vi "Coord window-FOV multiplier.vi"(11 "Absolute maximum coordinate":dbl) -> (3 "Field of view multiplier":sgl)   [LabVIEW 2013]
uses:
  <vilib>/gmath/NI_Gmath.lvlib
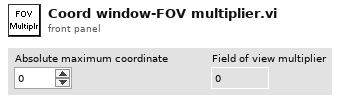
[diagram p1: front panel]
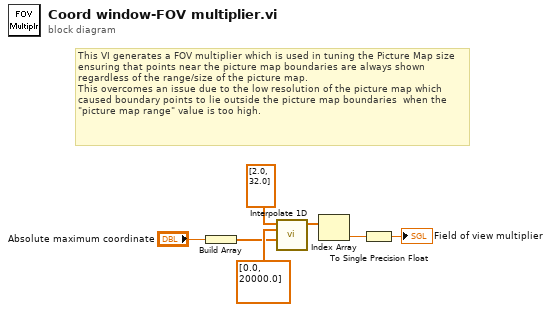
[diagram p0: block diagram]
diagram:
  # "This VI generates a FOV multiplier which is used in tuning the Picture Map size ensuring that points near the picture map boundaries are always shown regardless of the range/size of the picture map.\nThis overcomes an issue due to the low resolution of the picture map which caused boundary points to lie outside the picture map boundaries  when the \"picture map range\" value is too high."
  n1 = Build Array("Absolute maximum coordinate") -> (w4:dbl[])
  n2 = call <vilib>:"Interpolate 1D.vi"("xi"=w4, "X"=dbl[] [0.0, 20000.0] ("Y"), "Y"=dbl[] [2.0, 32.0]) -> ("yi"=w6:dbl[])  [unwired: 6 in, 2 out]
  n3 = Index Array(array=w6) -> (element=w7:dbl)  [unwired: 1 in]
  n4 = To Single Precision Float(number=w7) -> (single precision float=→"Field of view multiplier":sgl)
